vi "Defer Front Panel Update.vi"(8 "error in":errorcluster, 9 "Defer Panel Updates":bool, 11 "VI in":refnum<vi>) -> (0 "error out":errorcluster, 3 "VI out":refnum<vi>)   [LabVIEW 2021]
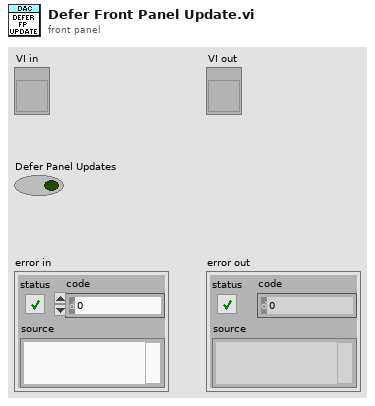
[diagram p1: front panel]
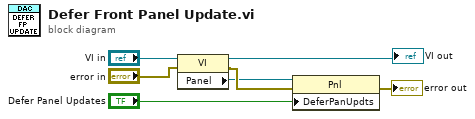
[diagram p0: block diagram]
diagram:
  n1 = property class="VI"(reference="VI in", error in="error in") -> (reference out=→"VI out":refnum<vi>, error out=w4:errorcluster, "Panel"=w2:refnum<vi>)
  n2 = property class="Pnl"(reference=w2, error in=w4, "DeferPanUpdts"="Defer Panel Updates") -> (error out=→"error out":errorcluster)  [unwired: 1 out]
